vi "InitGenerator.vi"(8 "error in (no error)":errorcluster, 10 "Generator ID in":T2 caption="RIO Device") -> (0 "error out":errorcluster, 1 "Init Done":bool, 2 "Waveform":cluster{"tv":dbl[], "DAC Codes":u16[]}, 3 "Generator ID out":T2, 4 "Generator Info":T1)   [LabVIEW 2018]
uses:
  <vilib>/userdefined/High Color/nirio_resource_hc.ctl
  Controls/GeneratorInfo.ctl
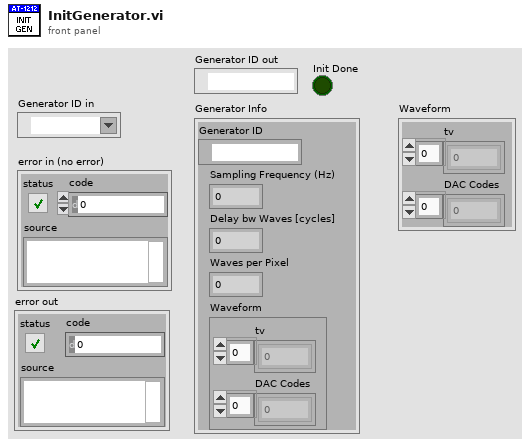
[diagram p1: front panel]
types:
  T1 = typedef "GeneratorInfo.ctl" = cluster{"Generator ID":T2, "Sampling Frequency (Hz)":u64, "Delay bw Waves [cycles]":u16, "Waves per Pixel":u32, "Waveform":cluster{"tv":dbl[], "DAC Codes":u16[]}}
  T2 = typedef "nirio_resource_hc.ctl" = tag
  T3 = cluster{"Generator ID in":T2, "Sampling Frequency (Hz)":u64, "Delay bw Waves [cycles]":u16, "Waves per Pixel":u32, "Waveform":cluster{"tv":dbl[], "DAC Codes":u16[]}}
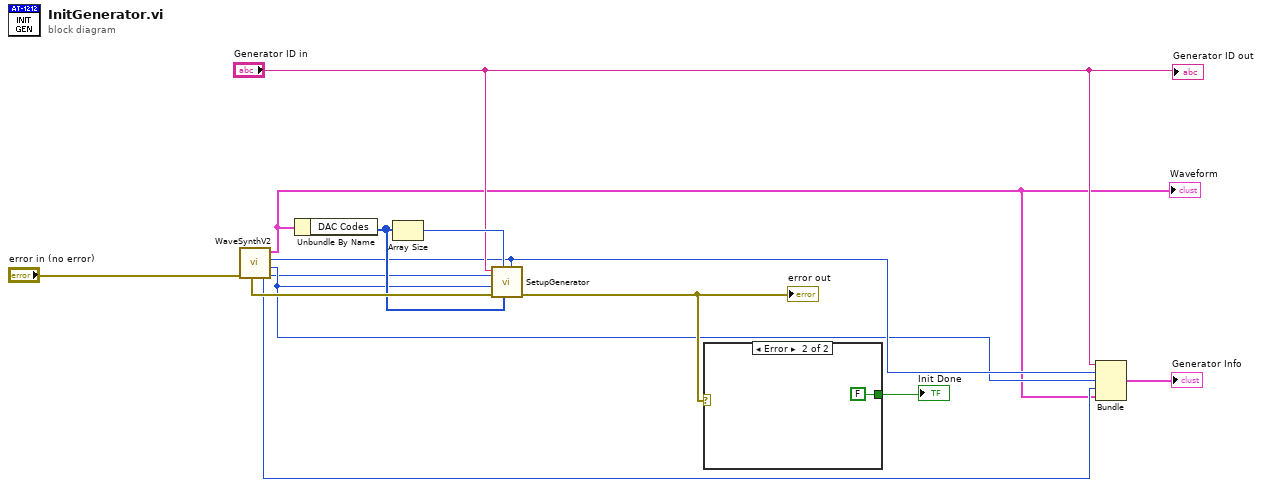
[diagram p0: block diagram]
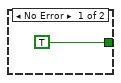
[diagram p2: hidden frame]
diagram:
  n1 = call "WaveSynthV2.vi"("error in"="error in (no error)") -> ("Waves per Pixel"=w3:u32, "Delay bw Waves [cycles]"=w4:u16, "Sampling Frequency (Hz)"=w5:u64, "Waveform"=w2:cluster{"tv":dbl[], "DAC Codes":u16[]}, "error out"=w12:errorcluster)  [unwired: 4 in]
  "Waveform" <- w2
  n2 = Unbundle By Name(w2) -> ("DAC Codes"=w10:u16[])
  n3 = Array Size(array=w10) -> (size(s)=w11:i32)
  n4 = call "SetupGenerator.vi"("Freq (Hz)"=w5, "DAC Codes"=w10, "NumSamples"=w11, "error in"=w12, "Delay bw waves [cycles]"=w4, "Waves Per Pixel"=w3, "RIO Device IN"="Generator ID in") -> ("error out"=w8:errorcluster)  [unwired: 4 in]
  "error out" <- w8
  n5 = case shown="Error" w8 {
    tunnel: [TRUE ("Init Done") FALSE ("Init Done")] -> w7
    frame No Error {
    }
    frame Error {
    }
  }
  "Init Done" <- w7
  n6 = Bundle("Generator ID in"="Generator ID in", "Sampling Frequency (Hz)"=w5, "Delay bw Waves [cycles]"=w4, "Waves per Pixel"=w3, "Waveform"=w2) -> (→"Generator Info":T3)  [unwired: 1 in]
  "Generator ID out" <- "Generator ID in"
